vi "DQMH_API_ArgumentWindow.vi"() -> ()   [LabVIEW 2014]
doc: "_____\nCreated using Delacor QMH Event Scripter 5.0.0.106."
panel:
  in  "EventArgument(String)":string
  # "Event Arguments Window"
  # "Instructions: Add controls to this panel. These controls will be added to the Arguments cluster for the new event. Use a descriptive label on each control.\n\nNote 1: There is no need to wrap the arguments with a cluster in this window. The Create New DQMH Event utility will take the controls in this VI and add them to an Arguments cluster when you are done. \n\nNote 2: If you are creating a Request and Wait for Reply event, you do not need to add the Notifier reference below... it will be created automatically.\n\nNote 3: If you are creating an event for a cloneable module, you do not need to add the Module ID control below... it will be created automatically."
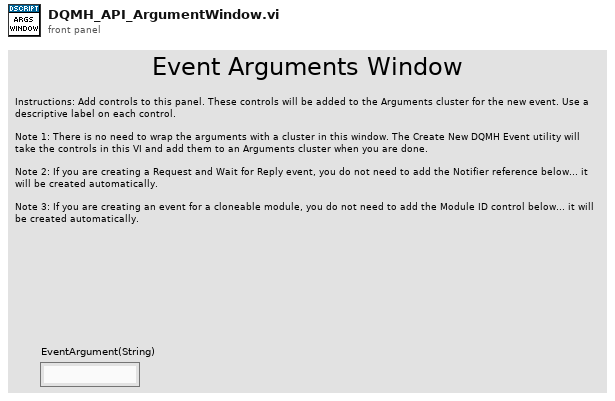
[diagram p1: front panel]
diagram:
